vi "TerminalExpression.vi"(8 "error in (no error)":errorcluster, 10 "data":string, 11 "TerminalExpression in":refnum<class "TerminalExpression.lvclass">) -> (0 "error out":errorcluster, 3 "TerminalExpression out":refnum<class "TerminalExpression.lvclass">)   [LabVIEW 2018, in "TerminalExpression.lvclass"]
uses:
  TerminalExpression.lvclass
  TerminalExpression.lvclass/TerminalExpression.ctl
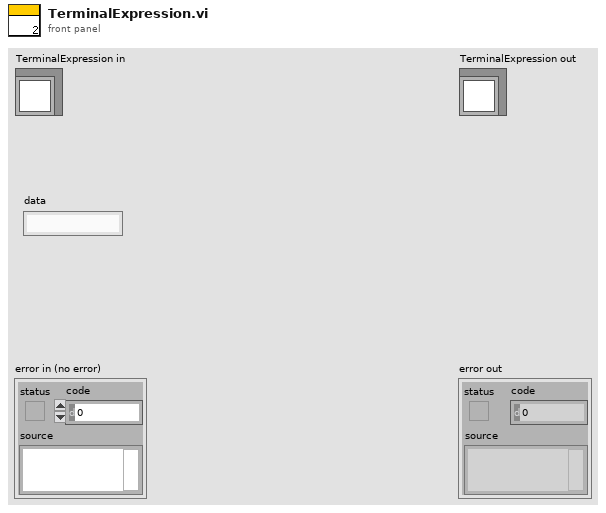
[diagram p1: front panel]
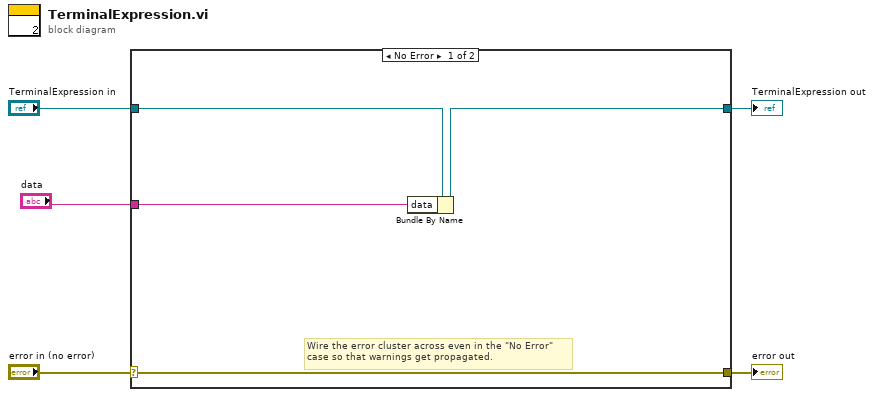
[diagram p0: block diagram]
diagram:
  n1 = case shown="No Error" "error in (no error)" {
    selector: "error in (no error)" -> [w8 w11]
    tunnel: [w8 w11] -> w4
    tunnel: [w7 w10] -> w2
    tunnel: "TerminalExpression in" -> [w9 w10]
    tunnel: "data" -> [w6 _]
    frame No Error {
      # "Wire the error cluster across even in the \"No Error\"\ncase so that warnings get propagated."
      n2 = Bundle By Name(cluster=w9, "data"=w6) -> (w7:refnum<class "TerminalExpression.lvclass">)
    }
    frame Error {
    }
  }
  "error out" <- w4
  "TerminalExpression out" <- w2
